vi "Plot Polar Data.vi"(4 "Size":u16, 5 "Legend Rectangle":T1, 6 "polar attributes":T3 {"minimum" format="%0.2f"; "maximum" format="%0.2f"}, 7 "grid measurements":T2 {"end angle" format="%0.2f"; "start angle" format="%0.2f"; "scale factors"."b" format="%0.2f"; "scale factors"."a" format="%0.2f"}, 8 "polar data":cluster{"magnitude":dbl, "phase":dbl}[](array[cluster]) {"phase" format="%0.2f"; "magnitude" format="%0.2f"}, 9 "picture":picture) -> (3 "new picture":picture)   [LabVIEW 2013]
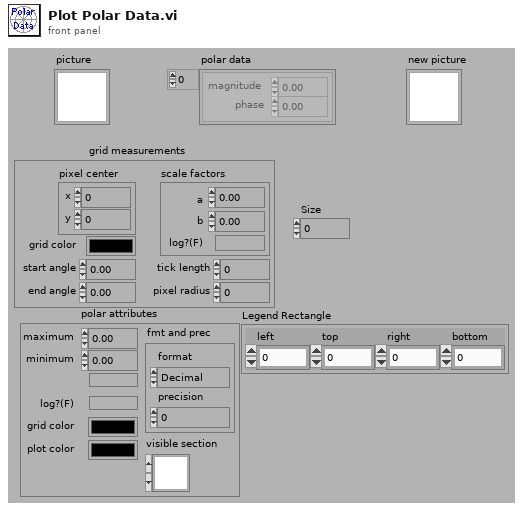
[diagram p1: front panel]
types:
  T1 = cluster{"left":i16, "top":i16, "right":i16, "bottom":i16}
  T2 = cluster{"pixel center":cluster{"x":i16, "y":i16}, "scale factors":cluster{"a":dbl, "b":dbl, "log?(F)":bool}, "grid color":u32, "start angle":dbl, "end angle":dbl, "tick length":i16, "pixel radius":i32}
  T3 = cluster{"maximum":dbl, "minimum":dbl, "clip to min":bool, "log?(F)":bool, "grid color":u32, "plot color":u32, "fmt and prec":cluster{"format":enum8{"Decimal", "Scientific", "Engineering", "Binary", "Octal", "Hex"}, "precision":u8}, "visible section":u16}
  T4 = cluster{"plot name":string, "plot color":u32, "fill?(F)":bool}
  T5 = enum32{"Solid", "Dash", "Dot", "DashDot", "DashDotDot"}
  T6 = cluster{"Size":u16, "Style":enum32{"Solid", "Dash", "Dot", "DashDot", "DashDotDot"}}
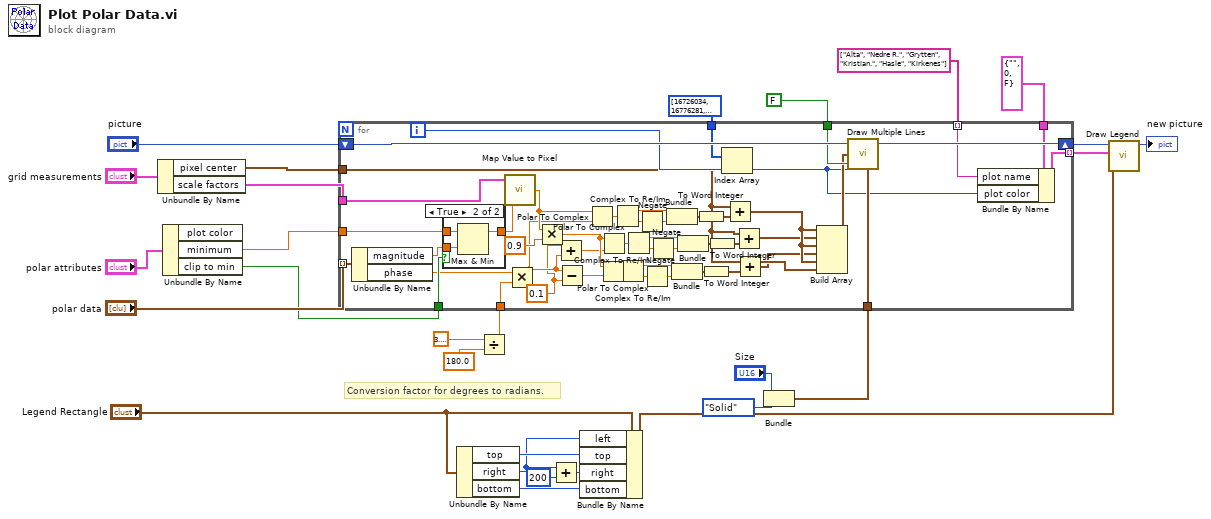
[diagram p0: block diagram]
diagram:
  # "Conversion factor for degrees to radians."
  n1 = Unbundle By Name("grid measurements") -> ("pixel center"=w24:cluster{"x":i16, "y":i16}, "scale factors"=w25:cluster{"a":dbl, "b":dbl, "log?(F)":bool})
  n2 = Unbundle By Name("polar attributes") -> ("minimum"=w23:dbl, "clip to min"=w22:bool)  [unwired: 1 out]
  n3 = Unbundle By Name("Legend Rectangle") -> ("top"=w5:i16, "right"=w2:i16, "bottom"=w4:i16)
  n4 = Divide(x=3.141592653589793, y=180.0) -> (x/y=w20:dbl)
  n5 = Add(x=w2, y=i16 200) -> (x+y=w3:i16)
  n6 = Bundle By Name(cluster="Legend Rectangle", "left"=w2, "top"=w5, "right"=w3, "bottom"=w4) -> (w6:T1)
  n7 = Bundle("Size"="Size", "Style"=T5."Solid") -> (w15:T6)  [unwired: 1 in]
  n8 = for {
    tunnel: "polar data" -> [w76] mode=indexing
    tunnel: w24 -> [w43]
    tunnel: w25 -> [w69]
    tunnel: w23 -> [w66]
    tunnel: w22 -> [w65]
    tunnel: w20 -> [w63]
    shift-right: [w61] -> w12
    shift-left: "picture" -> [w62]
    tunnel: w15 -> [w60]
    tunnel: FALSE -> [w59]
    tunnel: u32[] [16726034, 16776281, 65316, 2770175, 16722671, 16758082] ("Array") -> [w33]
    tunnel: T4 {"plot name"="", "plot color"=0, "fill?(F)"=FALSE} ("vi metric") -> [w32]
    tunnel: [w31] -> w9 mode=indexing
    tunnel: string[] ["Alta", "Nedre R.", "Grytten", "Kristian.", "Hasle", "Kirkenes"] -> [w29] mode=indexing
    i -> [w57]
    w34 = 0.1 ("x*y")
    n9 = Unbundle By Name(w76) -> ("magnitude"=w67:dbl, "phase"=w64:dbl)
    n10 = case shown="True" w65 {
      tunnel: w67 -> [w77 w80]
      tunnel: [w77 w79] -> w68
      tunnel: w66 -> [_ w78]
      frame False {
      }
      frame True {
        n11 = Max & Min(x=w78, y=w80) -> (max(x,y)=w79:dbl)  [unwired: 1 out]
      }
    }
    n12 = call <vilib>:"Map Value to Pixel.vi"("x"=w68, "scale factors"=w69) -> ("pixel"=w39:dbl)  [unwired: 1 out]
    n13 = Multiply(x=w64, y=w63) -> (x*y=w35:dbl)
    n14 = Multiply(x=w39, y=0.9 ("x*y")) -> (x*y=w40:dbl)
    n15 = Add(x=w34, y=w35) -> (x+y=w37:dbl)
    n16 = Subtract(x=w35, y=w34) -> (x-y=w36:dbl)
    n17 = Polar To Complex(1:w35, 2:w39) -> (0:w75:cdb)
    n18 = Polar To Complex(1:w36, 2:w40) -> (0:w50:cdb)
    n19 = Polar To Complex(1:w37, 2:w40) -> (0:w51:cdb)
    n20 = Complex To Re/Im(x + iy=w75) -> (x=w73:dbl, y=w72:dbl)
    n21 = Complex To Re/Im(x + iy=w50) -> (x=w48:dbl, y=w47:dbl)
    n22 = Complex To Re/Im(x + iy=w51) -> (x=w53:dbl, y=w54:dbl)
    n23 = Negate(x=w72) -> (-x=w70:dbl)
    n24 = Negate(x=w47) -> (-x=w46:dbl)
    n25 = Negate(x=w54) -> (-x=w55:dbl)
    n26 = Bundle(w73, w70) -> (w74:cluster{dbl, dbl})  [unwired: 1 out]
    n27 = Bundle(w48, w46) -> (w49:cluster{dbl, dbl})  [unwired: 1 out]
    n28 = Bundle(w53, w55) -> (w52:cluster{dbl, dbl})  [unwired: 1 out]
    n29 = To Word Integer(number=w74) -> (16bit integer=w71:cluster{i16, i16})
    n30 = To Word Integer(number=w49) -> (16bit integer=w44:cluster{i16, i16})
    n31 = To Word Integer(number=w52) -> (16bit integer=w45:cluster{i16, i16})
    n32 = Index Array(array=w33, index=w57) -> (element=w30:u32)
    n33 = Add(x=w43, y=w71) -> (x+y=w56:cluster{i16, i16})
    n34 = Add(x=w43, y=w45) -> (x+y=w41:cluster{i16, i16})
    n35 = Add(x=w43, y=w44) -> (x+y=w42:cluster{i16, i16})
    n36 = Build Array(w56, w41, w56, w42, w56, w43) -> (w58:cluster{"x":i16, "y":i16}[])
    n37 = call <vilib>:"Draw Multiple Lines.vi"("picture"=w62, "line endpoints"=w58, "fill?(F)"=w59, "color(black)"=w30, "pen"=w60) -> ("new picture"=w61:picture)  [unwired: 4 out]
    n38 = Bundle By Name(cluster=w32, "plot name"=w29, "plot color"=w30) -> (w31:T4)
  }
  n39 = call <vilib>:"Draw Legend.vi"("rect"=w6, "plot info"=w9, "picture"=w12) -> ("new picture"=→"new picture":picture)  [unwired: 8 in]
